vi "StringArrayIntersection.vi"(10 "Fewer":string[](array[string]), 11 "More":string[](array[string])) -> (3 "Intersection":string[](array[string]))   [LabVIEW 2019]
uses:
  16bd730e-c6ec-40f3-b56c-7a2d952d1711.vi
  3c22b8b1-0670-400c-b7c7-0996c59c043d.vi
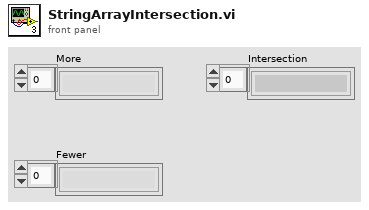
[diagram p1: front panel]
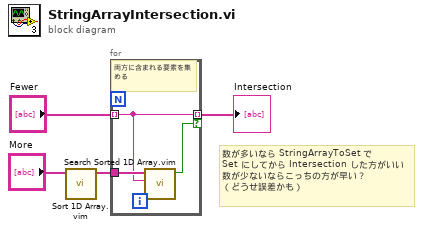
[diagram p0: block diagram]
diagram:
  # "数が多いなら StringArrayToSet で\nSet にしてから Intersection した方がいい\n数が少ないならこっちの方が早い？\n（どうせ誤差かも）"
  n1 = call "Sort 1D Array.vim"("unsorted array"="More") -> ("sorted array"=w2:string[])  [unwired: 10 in]
  n2 = for {
    tunnel: w2 -> [w7]
    tunnel: "Fewer" -> [w6] mode=indexing
    tunnel: [w6] -> w4 mode=indexing if=w5
    # "両方に含まれる要素を集める"
    n3 = call "Search Sorted 1D Array.vim"("element"=w6, "sorted 1D array"=w7) -> ("found?"=w5:bool)  [unwired: 8 in, 1 out]
  }
  "Intersection" <- w4
